vi "OneSessTwoPinOneInstrOneSiteReservation_CallNiDcPowerGetConnections1Pin1Connection_ReturnsOneConnection.vi"(8 "error in":errorcluster) -> (0 "error out":errorcluster, 2 "result":string, 3 "pass":bool)   [LabVIEW 2020, in "MeasurementServerTests.lvlib"]
uses:
  MeasurementServerTests.lvlib
  Runtime/MeasurementLink Session Management/Session Reservation/Connection.ctl
  Runtime/MeasurementLink Session Management/Session Reservation/Session Reservation.lvclass
  b3e5c3be-b7a7-4b6e-86ee-709eea9cb752.vi
  03fc85e1-696b-4ece-a78b-f41470766ac0.vi
  Runtime/MeasurementLink niDCPower/MeasurementLink niDCPower.lvlib
  Runtime/MeasurementLink niDCPower/Connection with Session.ctl
  Runtime/MeasurementLink niDCPower/Get Connections - 1Pin 1Conn.vi
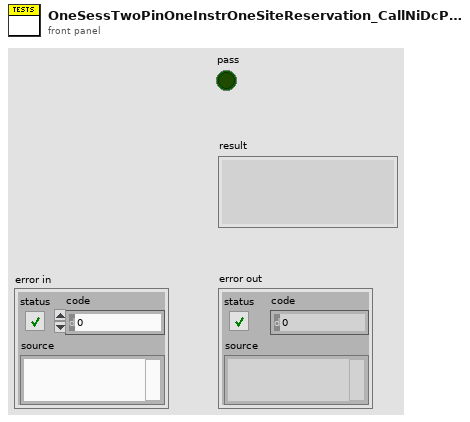
[diagram p1: front panel]
types:
  T1 = typedef "MeasurementLink niDCPower.lvlib/Connection with Session.ctl" = cluster{"connection":T2, "session":refnum<k15>}
  T2 = typedef "MeasurementLink Session Management.lvlib/Session Reservation.lvclass/Connection.ctl" = cluster{"pin or relay name":string, "site":i32, "instrument type id":string, "channel":string}
  T3 = typedef "MeasurementLink Session Management.lvlib/Session Reservation.lvclass/Data.ctl" = cluster{"session and driver infos":T4[], "pin or relay names":string[]}
  T4 = typedef "MeasurementLink Session Management.lvlib/Session Reservation.lvclass/Session and Driver Info.ctl" = cluster{"session info":T5, "session":variant}
  T5 = typedef "MeasurementLink Session Management Client.lvlib/ni_measurementlink_sessionmanagement_v1_SessionInformation.ctl" = cluster{"session":T6, "resource_name":string, "channel_list":string, "instrument_type_id":string, "session_exists":bool, "channel_mappings":T7[]}
  T6 = typedef "MeasurementLink Session Management Client.lvlib/nidevice_grpc_Session.ctl" = cluster{"name":string}
  T7 = typedef "MeasurementLink Session Management Client.lvlib/ni_measurementlink_sessionmanagement_v1_ChannelMapping.ctl" = cluster{"pin_or_relay_name":string, "site":i32, "channel":string}
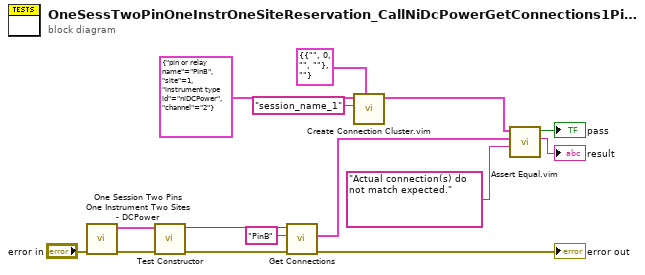
[diagram p0: block diagram]
diagram:
  n1 = call "One Session Two Pins One Instrument Two Sites - DCPower.vi"("error in"="error in") -> ("error out"=w8:errorcluster, "data out"=w7:T3)  [unwired: 9 in]
  n2 = call "Test Constructor.vi"("error in"=w8, "data"=w7) -> ("error out"=w15:errorcluster, "Session Reservation out"=w14:refnum<class "Session Reservation.lvclass">)  [unwired: 8 in]
  n3 = call-poly "Get Connections.vi"("error in"=w15, "pin or relay name"="PinB", "session reservation in"=w14) -> ("error out"=→"error out":errorcluster, "connection"=w12:T1)  [unwired: 6 in, 1 out]
  n4 = call "Create Connection Cluster.vim"("connection type"=T1 {"connection"={"pin or relay name"="", "site"=0, "instrument type id"="", "channel"=""}, "session"=""} ("niDCPower connection"), "session in"="session_name_1", "hardware independent connection in"=T2 {"pin or relay name"="PinB", "site"=1, "instrument type id"="niDCPower", "channel"="2"} ("connection")) -> ("connection out"=w6:T1)  [unwired: 8 in]
  n5 = call "Assert Equal.vim"("failure message"="Actual connection(s) do not match expected.", "actual value"=w12, "expected value"=w6) -> ("message"=→"result":string, "equal?"=→"pass":bool)  [unwired: 7 in]
